vi "testEnumFormatting.vi"(8 "error in (no error)":errorcluster, 11 "reference in":refnum<class "EasyXMLTest.lvclass">) -> (0 "error out":errorcluster, 3 "reference in":refnum<class "EasyXMLTest.lvclass">)   [LabVIEW 2011, in "EasyXMLTest.lvclass"]
uses:
  EasyXMLTest.lvclass
  <vilib>/addons/_JKI Toolkits/VI Tester/TestCase.llb/TestCase.lvclass
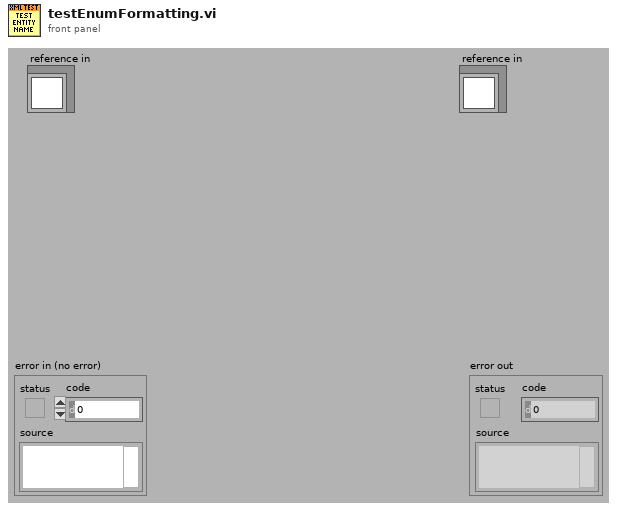
[diagram p1: front panel]
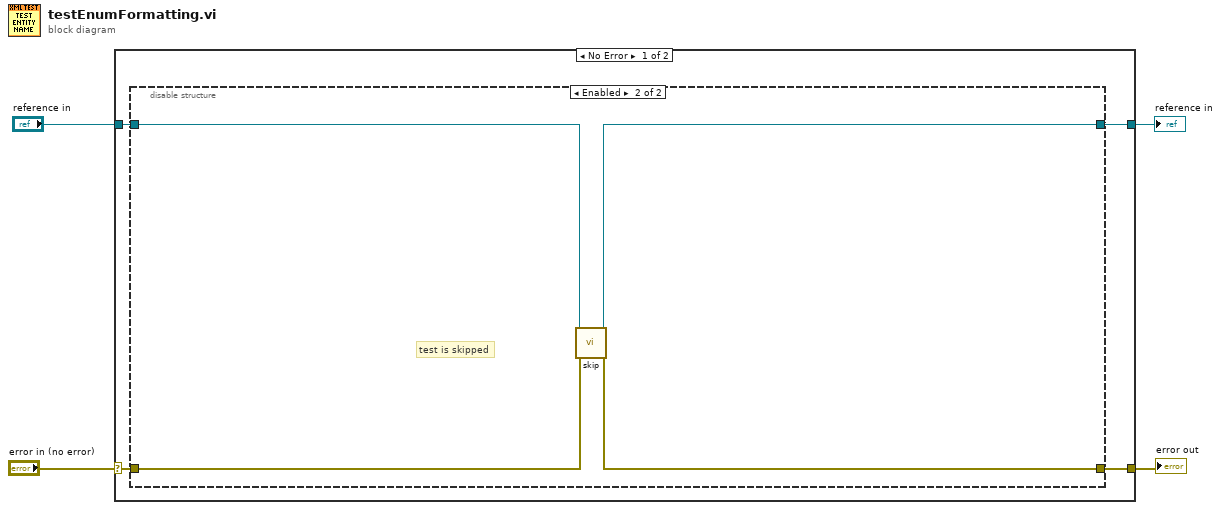
[diagram p0: block diagram]
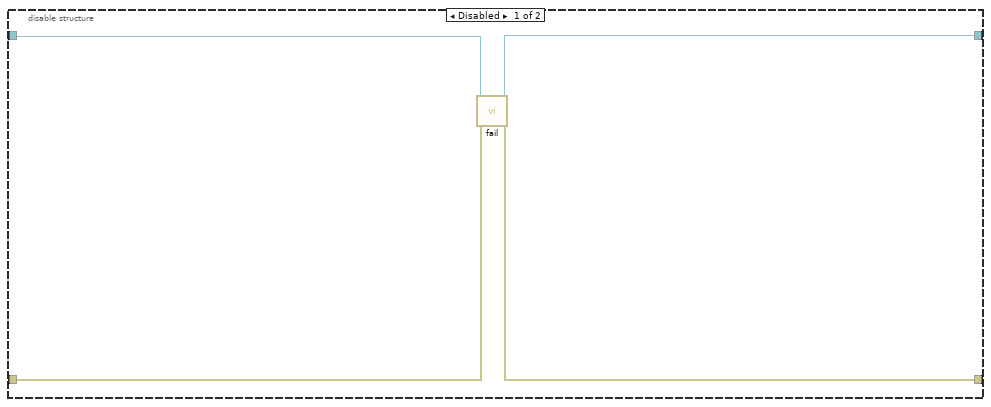
[diagram p2: hidden frame]
diagram:
  n1 = case shown="No Error" "error in (no error)" {
    selector: "error in (no error)" -> [w7 w18]
    tunnel: [w5 w18] -> w3
    tunnel: [w6 w17] -> w1
    tunnel: "reference in" -> [w8 w17]
    frame No Error {
      n2 = disable-structure shown="Enabled" {
        disable-tunnel: w8 -> [w12 w16]
        disable-tunnel: w7 -> [w9 w14]
        disable-tunnel: [w11 w15] -> w6
        disable-tunnel: [w10 w13] -> w5
        frame Disabled {
          n3 = call-dynamic "fail.vi"("error in (no error)"=w9, "TestCase in"=w12) -> ("error out"=w10:errorcluster, "TestCase out"=w11:refnum<class "EasyXMLTest.lvclass">)  [unwired: 8 in]
        }
        frame Enabled {
          # "test is skipped"
          n4 = call <vilib>:"skip.vi"("error in (no error)"=w14, "TestCase in"=w16) -> ("error out"=w13:errorcluster, "TestCase out"=w15:refnum<class "EasyXMLTest.lvclass">)  [unwired: 8 in]
        }
      }
    }
    frame Error {
    }
  }
  "error out" <- w3
  "reference in" <- w1
